vi "get log status.vi"(8 "error in (no error)":errorcluster) -> (0 "error out":errorcluster, 3 "active":bool)   [LabVIEW 2024, in "atsj peakcan basic.lvlib"]
uses:
  atsj peakcan basic.lvlib
  parameter.ctl
  get parameter - i32.vi
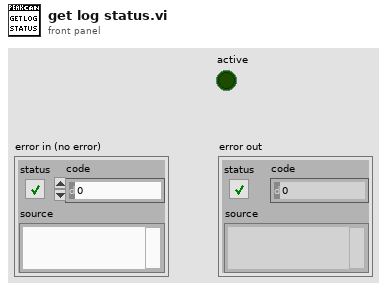
[diagram p1: front panel]
types:
  T1 = typedef "atsj peakcan basic.lvlib/parameter.ctl" = enum8{"DEVICE_ID", "5VOLTS_POWER", "RECEIVE_EVENT", "MESSAGE_FILTER", "API_VERSION", "CHANNEL_VERSION", "BUSOFF_AUTORESET", "LISTEN_ONLY", "LOG_LOCATION", "LOG_STATUS", "LOG_CONFIGURE", "LOG_TEXT", "CHANNEL_CONDITION", "HARDWARE_NAME", "RECEIVE_STATUS", "CONTROLLER_NUMBER", "TRACE_LOCATION", "TRACE_STATUS", "TRACE_SIZE", "TRACE_CONFIGURE", "CHANNEL_IDENTIFYING", "CHANNEL_FEATURES", "BITRATE_ADAPTING", "BITRATE_INFO", "BITRATE_INFO_FD", "BUSSPEED_NOMINAL", "BUSSPEED_DATA", "IP_ADDRESS", "LAN_SERVICE_STATUS", "ALLOW_STATUS_FRAMES", "ALLOW_RTR_FRAMES", "ALLOW_ERROR_FRAMES", "INTERFRAME_DELAY", "ACCEPTANCE_FILTER_11BIT", "ACCEPTANCE_FILTER_29BIT", "IO_DIGITAL_CONFIGURATION", "IO_DIGITAL_VALUE", "IO_DIGITAL_SET", "IO_DIGITAL_CLEAR", "IO_ANALOG_VALUE", "FIRMWARE_VERSION", "ATTACHED_CHANNELS_COUNT", "ATTACHED_CHANNELS", "ALLOW_ECHO_FRAMES", "DEVICE_PART_NUMBER", "HARD_RESET_STATUS", "LAN_CHANNEL_DIRECTION", "DEVICE_GUID"}
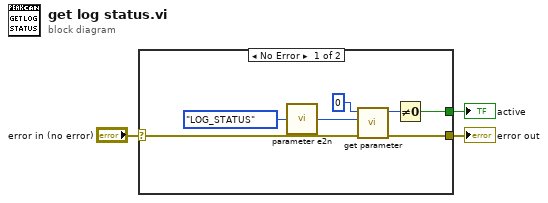
[diagram p0: block diagram]
diagram:
  n1 = case shown="No Error" "error in (no error)" {
    selector: "error in (no error)" -> [w7 w11]
    tunnel: [w6 w11] -> w1
    tunnel: [w4 _] -> w2
    frame No Error {
      n2 = call "parameter e2n.vi"("parameter"=parameter."LOG_STATUS") -> ("number"=w8:u8)
      n3 = call-poly "get parameter.vi"("error in (no error)"=w7, "parameter"=w8, "channel"=u16 0) -> ("error out"=w6:errorcluster, "value"=w5:i32)  [unwired: 7 in]
      n4 = Not Equal To 0?(x=w5) -> (x != 0?=w4:bool)
    }
    frame Error {
    }
  }
  "active" <- w2
  "error out" <- w1
